vi "AttrMap-Probe.vi"(11 "AttrMap out":T1) -> (2 "Value String":string, 3 "Boolean":bool)   [LabVIEW 2019]
uses:
  Typedef/Def-AttrMap.ctl
panel:
  in  "Tree":string(tree)
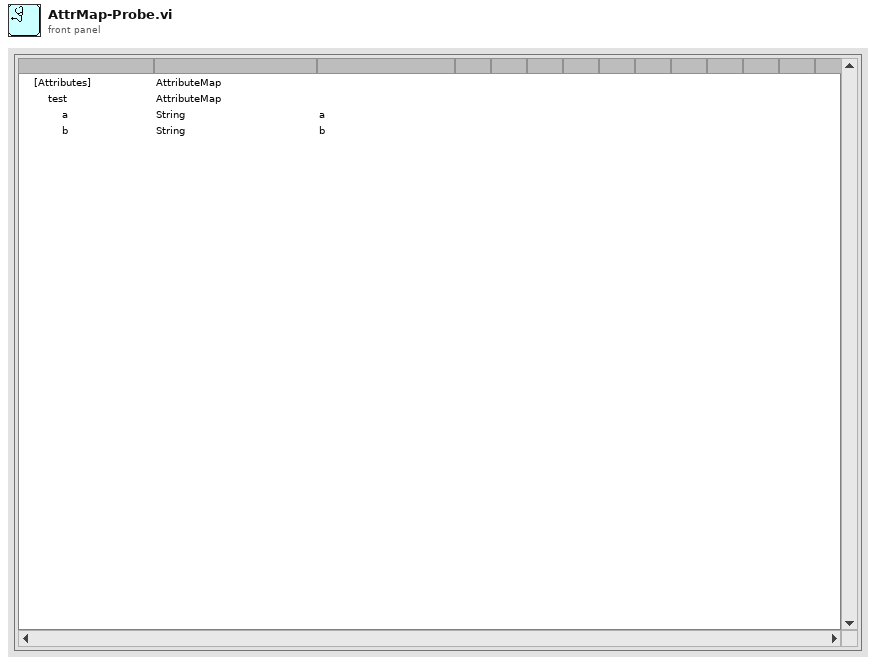
[diagram p1: front panel]
types:
  T1 = typedef "Def-AttrMap.ctl" = cluster{"Map":variant}
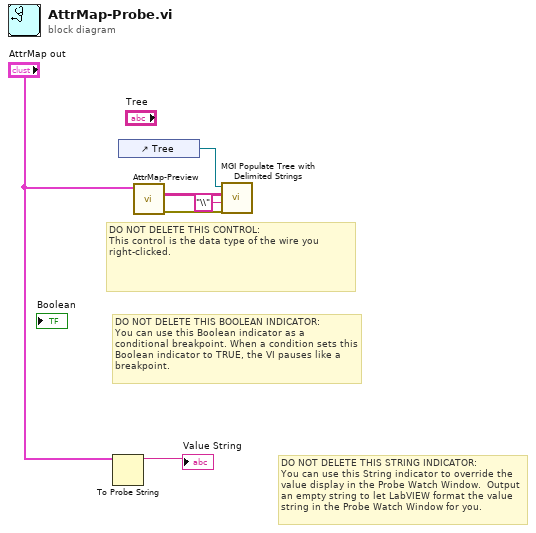
[diagram p0: block diagram]
diagram:
  # "DO NOT DELETE THIS STRING INDICATOR: \nYou can use this String indicator to override the value display in the Probe Watch Window.  Output an empty string to let LabVIEW format the value string in the Probe Watch Window for you."
  # "DO NOT DELETE THIS BOOLEAN INDICATOR: \nYou can use this Boolean indicator as a conditional breakpoint. When a condition sets this Boolean indicator to TRUE, the VI pauses like a breakpoint."
  # "DO NOT DELETE THIS CONTROL: \nThis control is the data type of the wire you right-clicked."
  n1 = To Probe String(7:"AttrMap out") -> (3:→"Value String":string)  [unwired: 2 in, 1 out]
  n2 = control-ref of="Tree"() -> (w4:refnum<vi>)
  n3 = call "AttrMap-Preview.vi"("AttrMap in"="AttrMap out") -> ("error out"=w5:errorcluster, "table"=w3:string[][])  [unwired: 8 in, 1 out]
  n4 = call <userlib>:"MGI Populate Tree with Delimited Strings.vi"("error in (no error)"=w5, "Delimiter"="\\", "Items (Delimited)"=w3, "Tree Control"=w4) -> ()  [unwired: 5 in, 3 out]
